vi "StopStreaming.vi"(8 "error in (no error)":errorcluster, 11 "CameraTestingProxy in":refnum<class "CameraTestingProxyAPI.lvclass">) -> (0 "error out":errorcluster, 3 "CameraTestingProxy out":refnum<class "CameraTestingProxyAPI.lvclass">)   [LabVIEW 2020, in "CameraTestingProxy.lvlib" / "CameraTestingProxyAPI.lvclass"]
uses:
  CameraTestingProxyAPI.lvclass
  db9ea65e-981f-4e8e-91cf-3c8e6b443aa0.vi
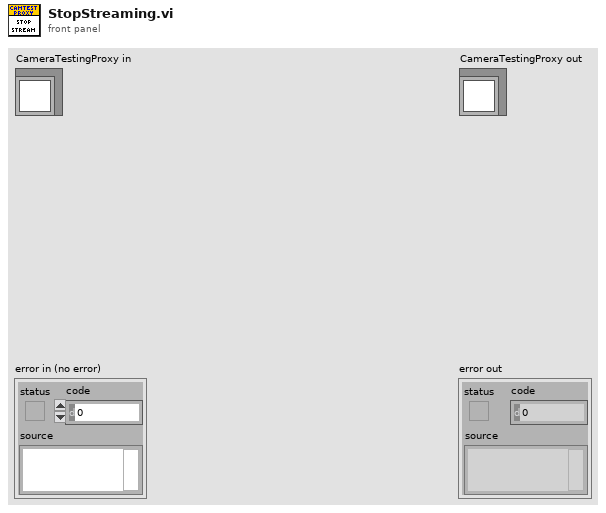
[diagram p1: front panel]
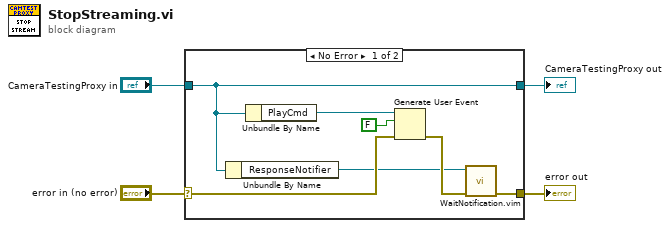
[diagram p0: block diagram]
diagram:
  n1 = case shown="No Error" "error in (no error)" {
    selector: "error in (no error)" -> [w10 w13]
    tunnel: [w7 w13] -> w1
    tunnel: [w6 w12] -> w3
    tunnel: "CameraTestingProxy in" -> [w6 w12]
    frame No Error {
      n2 = Unbundle By Name(w6) -> ("ResponseNotifier"=w5:refnum<notifier>)
      n3 = Unbundle By Name(w6) -> ("PlayCmd"=w11:refnum<user-event>)
      n4 = Generate User Event(user event=w11, event data cluster=FALSE ("event data"), error in=w10) -> (error out=w8:errorcluster)  [unwired: 1 in, 1 out]
      n5 = call "WaitNotification.vim"("error in (no error)"=w8, "ResponseNotifier"=w5) -> ("error out"=w7:errorcluster)  [unwired: 8 in, 1 out]
    }
    frame Error {
    }
  }
  "error out" <- w1
  "CameraTestingProxy out" <- w3
